vi "LWConvertArrayIntoDotNetList.vi"(8 "Error IN":errorcluster, 11 "array of axes":i32[](array[numeric])) -> (0 "Error OUT":errorcluster, 3 "\"axes\" List":refnum<k24>)   [LabVIEW 2015]
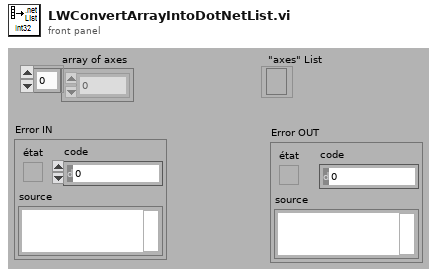
[diagram p1: front panel]
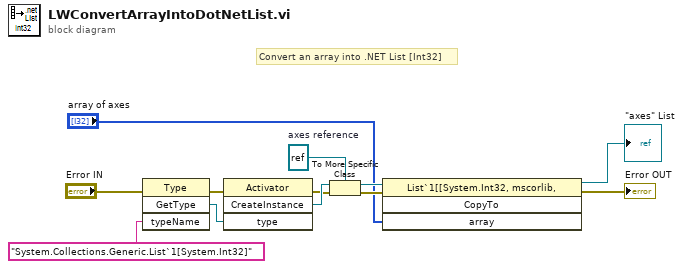
[diagram p0: block diagram]
diagram:
  w8 = refnum<k24> refnum  # axes reference
  # "Convert an array into .NET List [Int32]"
  n1 = invoke class="Type" method="GetType"(error in="Error IN", "typeName"="System.Collections.Generic.List`1[System.Int32]") -> (error out=w9:errorcluster, "GetType"=w10:refnum<k24>)  [unwired: 2 in, 2 out]
  n2 = invoke class="Activator" method="CreateInstance"(error in=w9, "type"=w10) -> (error out=w11:errorcluster, "CreateInstance"=w12:refnum<k24>)  [unwired: 2 in, 2 out]
  n3 = To More Specific Class(target class=w8, reference=w12, error in=w11) -> (specific class reference=w7:refnum<k24>, error out=w6:errorcluster)
  n4 = invoke class="List`1[[System.Int32, mscorlib," method="CopyTo"(reference=w7, error in=w6, "array"="array of axes") -> (reference out=→"\"axes\" List":refnum<k24>, error out=→"Error OUT":errorcluster)  [unwired: 1 in, 2 out]
